vi "CLD 12 Timer.vi"(8 "Error In":errorcluster, 10 "Time Target (s)":dbl, 11 "CLD 12 Timer Enum":T1) -> (0 "Error Out":errorcluster, 2 "Has Time Elapsed ?":bool, 3 "Elapsed Time (s.ss)":dbl)   [LabVIEW 2009]
doc: "CLD 12 Exercise\n\nThis VI is used as a FGV. The Reset Timer state uses the current time target, the Start Timer state reads a new time target from the caller.\n\n\n\n\n\nNote on reading time when in pause. The developer should not call the read time function when in pause; however, a case structure is used to defensively program the read state for this possibility."
uses:
  CLD12 Timer Enum.ctl
panel:
  out "Elapsed Time (s)":dbl
  out "Elapsed Time (s.sssss)":dbl
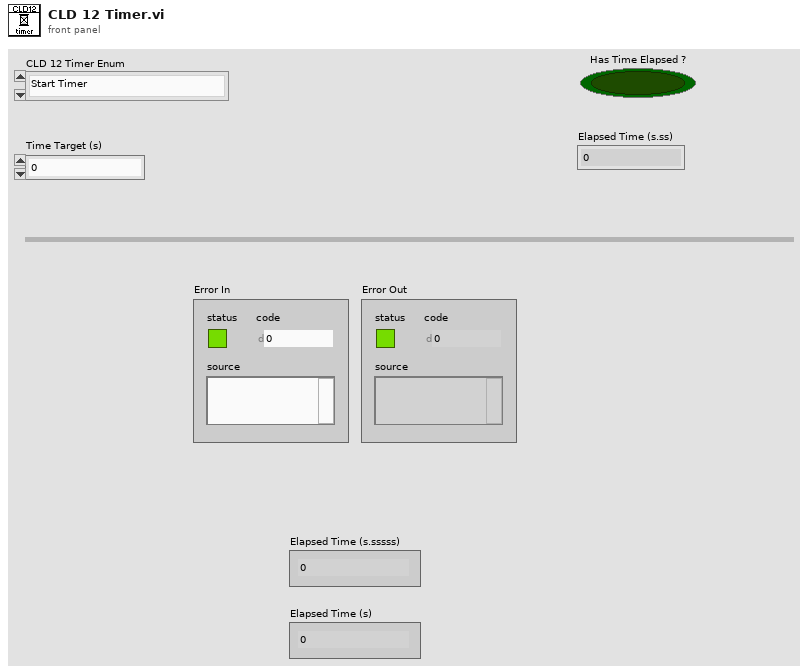
[diagram p1: front panel]
types:
  T1 = typedef "CLD12 Timer Enum.ctl" = enum16{"Start Timer", "Read Time", "Pause", "UnPause", "Reset Timer"}
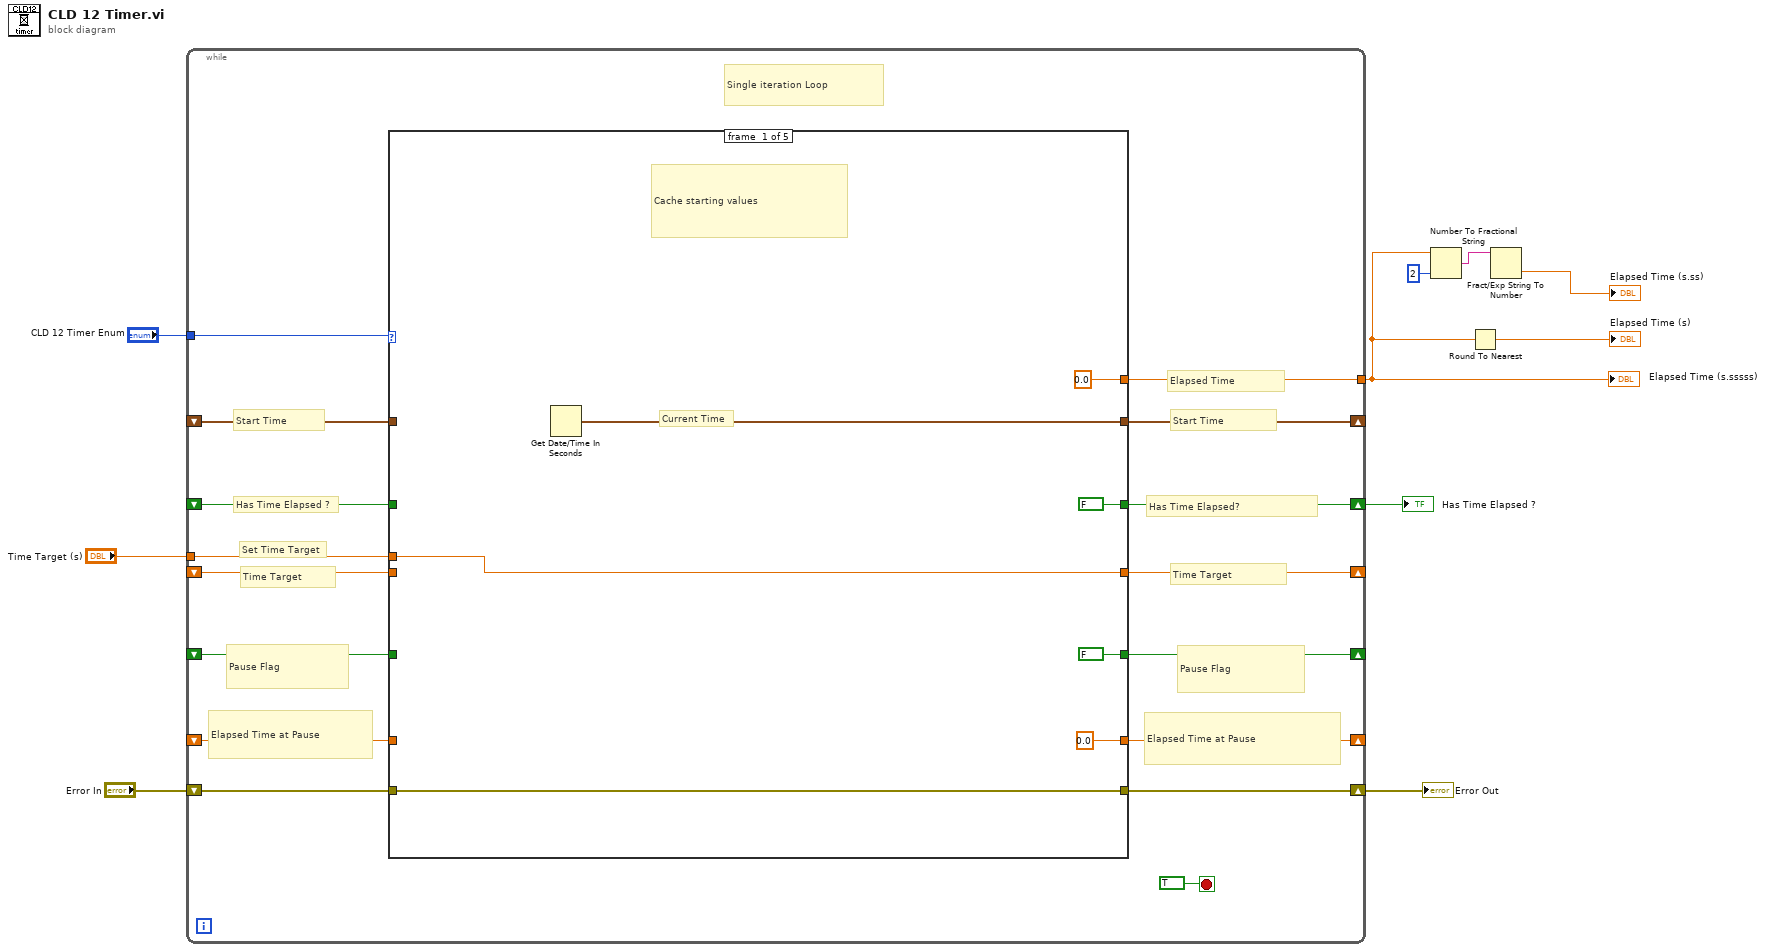
[diagram p0: block diagram]
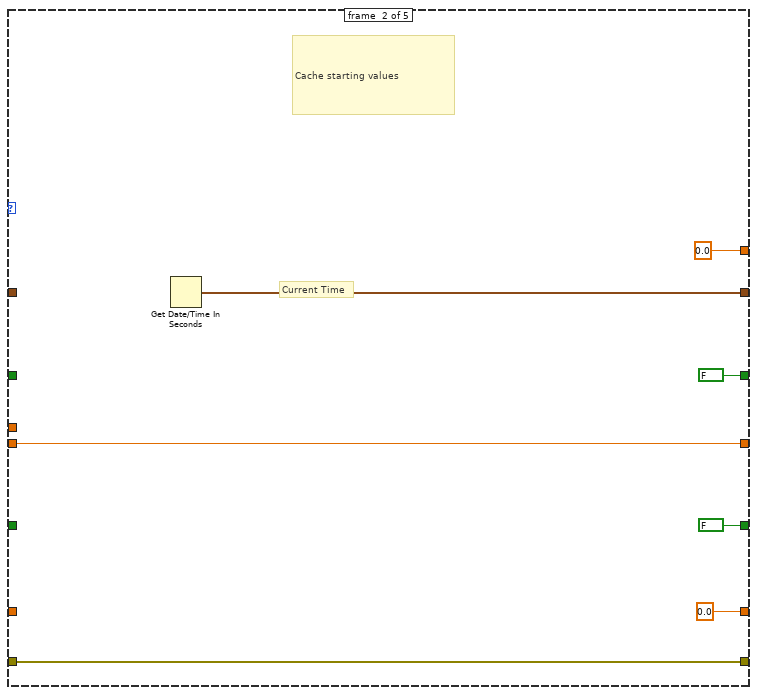
[diagram p2: hidden frame]
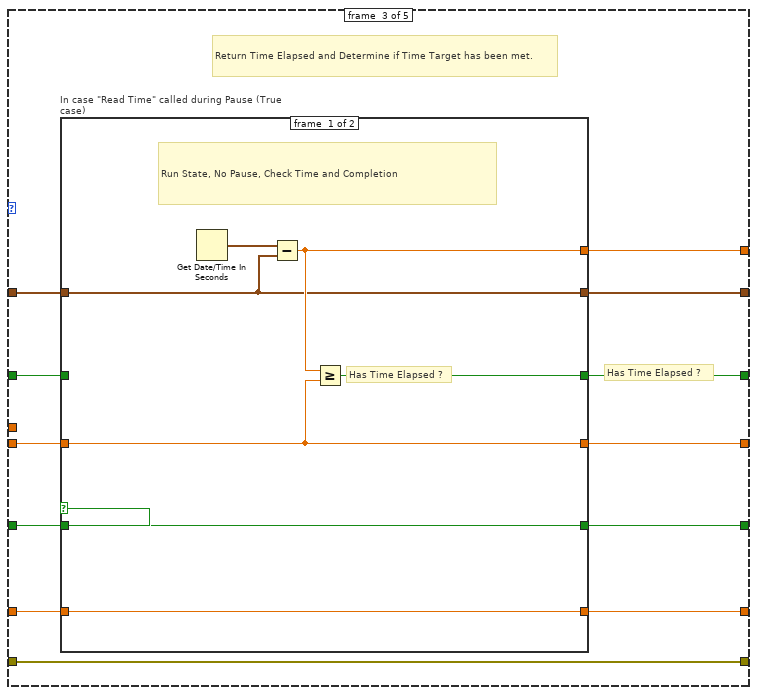
[diagram p3: hidden frame]
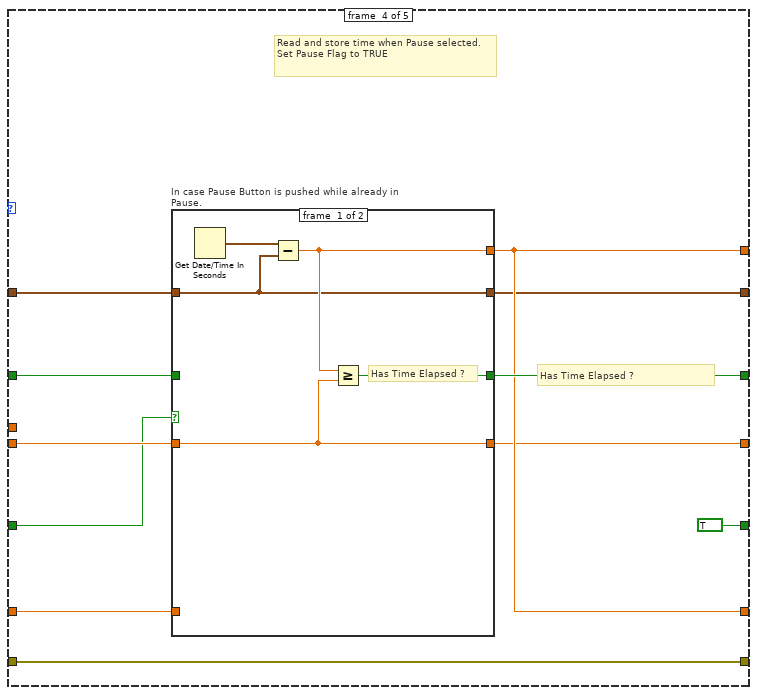
[diagram p5: hidden frame]
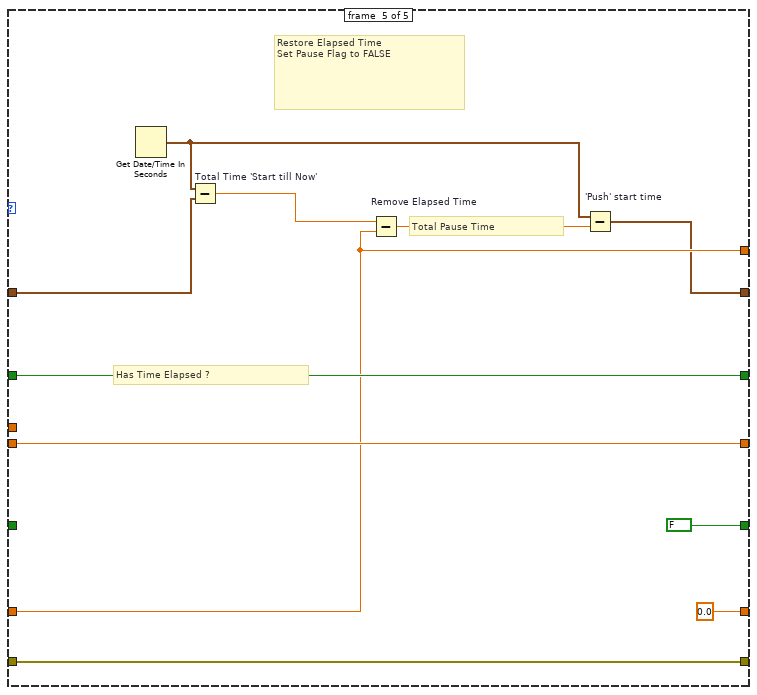
[diagram p7: hidden frame]
diagram:
  n1 = while {
    tunnel: "CLD 12 Timer Enum" -> [w26]
    shift-right: [w24] -> _
    shift-left: _ -> [w23]
    tunnel: [w22] -> w4
    shift-right: [w21] -> w9
    shift-left: "Error In" -> [w20]
    tunnel: "Time Target (s)" -> [w17]
    shift-right: [w18] -> _
    shift-left: _ -> [w19]
    shift-right: [w16] -> w6
    shift-left: _ -> [w15]
    shift-right: [w14] -> _
    shift-left: _ -> [w13]
    shift-right: [w12] -> _
    shift-left: _ -> [w11]
    stop <- TRUE ("stop") stop-if-true
    # "Start Time"
    # "Start Time"
    # "Elapsed Time"
    # "Time Target"
    # "Time Target"
    # "Set Time Target"
    # "Has Time Elapsed?"
    # "Has Time Elapsed ?"
    # "Pause Flag"
    # "Pause Flag"
    # "Elapsed Time at Pause"
    # "Elapsed Time at Pause"
    # "Single iteration Loop"
    n2 = case shown="\"UnPause\"" w26 {
      tunnel: [w33 w40 w44 w64 w84] -> w24
      tunnel: w23 -> [_ _ w51 w74 w89]
      tunnel: [0.0 ("Elapsed Time") 0.0 ("Elapsed Time") w47 w69 w87] -> w22
      tunnel: [w31 w38 w50 w73 w94] -> w21
      tunnel: w20 -> [w31 w38 w50 w73 w94]
      tunnel: w19 -> [_ w34 w49 w72 w93]
      tunnel: [w27 w34 w49 w65 w93] -> w18
      tunnel: w17 -> [w27 _ _ _ _]
      tunnel: [FALSE FALSE w48 w71 w91] -> w16
      tunnel: w15 -> [_ _ w41 w68 w91]
      tunnel: [FALSE FALSE w43 TRUE FALSE] -> w14
      tunnel: w13 -> [_ _ w42 w67 _]
      tunnel: [0.0 0.0 w45 w69 0.0] -> w12
      tunnel: w11 -> [_ _ w46 w66 w87]
      frame #0 {
        # "Current Time"
        # "Cache starting values"
        n3 = Get Date/Time In Seconds() -> (seconds since 1Jan1904=w33:timestamp)
      }
      frame #1 {
        # "Current Time"
        # "Cache starting values"
        n4 = Get Date/Time In Seconds() -> (seconds since 1Jan1904=w40:timestamp)
      }
      frame #2 {
        # "Has Time Elapsed ?"
        # "Return Time Elapsed and Determine if Time Target has been met."
        n5 = case "In case \"Read Time\" called during Pause (True case)" shown="False" w42 {
          tunnel: w51 -> [w55 w63]
          tunnel: w49 -> [w54 w62]
          tunnel: [w57 w60] -> w48
          tunnel: [w56 w59] -> w47
          tunnel: w46 -> [w52 w59]
          tunnel: [w52 w59] -> w45
          tunnel: [w55 w63] -> w44
          tunnel: [w54 w62] -> _
          tunnel: [w53 w61] -> w43
          tunnel: w42 -> [w53 w61]
          tunnel: w41 -> [_ w60]
          frame #0 {
            # "Has Time Elapsed ?"
            # "Run State, No Pause, Check Time and Completion"
            n6 = Get Date/Time In Seconds() -> (seconds since 1Jan1904=w58:timestamp)
            n7 = Subtract(x=w58, y=w55) -> (x-y=w56:dbl)
            n8 = Greater Or Equal?(x=w56, y=w54) -> (x >= y?=w57:bool)
          }
          frame #1 {
            # "Pause State, Just return Shift Registers. Do not call 'Read Time'  when in pause."
          }
        }
      }
      frame #3 {
        # "Has Time Elapsed ?"
        # "Read and store time when Pause selected.\nSet Pause Flag to TRUE"
        n9 = case "In case Pause Button is pushed while already in Pause." shown="False" w67 {
          tunnel: w74 -> [w75 w80]
          tunnel: w72 -> [w76 w81]
          tunnel: [w78 w83] -> w71
          tunnel: [w77 w82] -> w69
          tunnel: w68 -> [_ w83]
          tunnel: w66 -> [_ w82]
          tunnel: [w76 w81] -> w65
          tunnel: [w75 w80] -> w64
          frame #0 {
            # "Has Time Elapsed ?"
            n10 = Get Date/Time In Seconds() -> (seconds since 1Jan1904=w79:timestamp)
            n11 = Subtract(x=w79, y=w75) -> (x-y=w77:dbl)
            n12 = Greater Or Equal?(x=w77, y=w76) -> (x >= y?=w78:bool)
          }
          frame #1 {
            # "Pause called when already in pause.\n\nJust read the registers and pass out the values."
          }
        }
      }
      frame #4 {
        # "Has Time Elapsed ?"
        # "Total Pause Time"
        # "Restore Elapsed Time\nSet Pause Flag to FALSE"
        n13 = Get Date/Time In Seconds() -> (seconds since 1Jan1904=w86:timestamp)
        n14 = Subtract "Total Time 'Start till Now'"(x=w86, y=w89) -> (x-y=w88:dbl)
        n15 = Subtract "Remove Elapsed Time"(x=w88, y=w87) -> (x-y=w85:dbl)
        n16 = Subtract "'Push' start time"(x=w86, y=w85) -> (x-y=w84:timestamp)
      }
    }
  }
  "Elapsed Time (s.sssss)" <- w4
  "Error Out" <- w9
  "Has Time Elapsed ?" <- w6
  n17 = Number To Fractional String(number=w4, precision (6)=i16 2) -> (F-format string=w3:string)  [unwired: 2 in]
  n18 = Round To Nearest(number=w4) -> (nearest integer value=→"Elapsed Time (s)":dbl)
  n19 = Fract/Exp String To Number(string=w3) -> (number=→"Elapsed Time (s.ss)":dbl)  [unwired: 3 in, 1 out]
